vi "py-lv-comm_readInt.vi"(7 "Property":bool, 8 "error in (no error)":errorcluster, 9 "arguments":string[](array[string]), 10 "function":string, 11 "zmq_socket in":refnum<class "zmq_socket.lvclass">) -> (0 "error out":errorcluster, 2 "int result":i32, 3 "zmq_socket out":refnum<class "zmq_socket.lvclass">)   [LabVIEW 2016]
uses:
  <vilib>/addons/zeromq/zmq_socket.lvclass
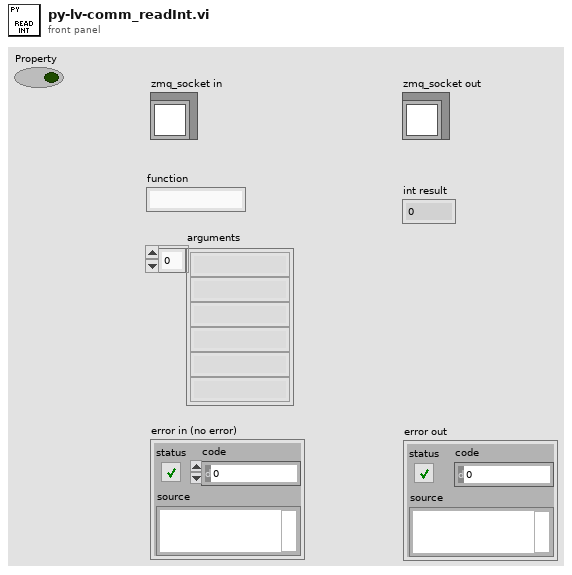
[diagram p1: front panel]
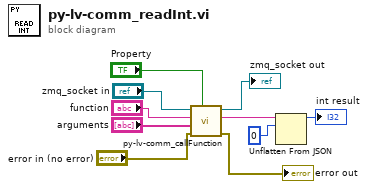
[diagram p0: block diagram]
diagram:
  n1 = call "py-lv-comm_callFunction.vi"("Property (F)"="Property", "error in (no error)"="error in (no error)", "arguments"="arguments", "function"="function", "zmq_socket in"="zmq_socket in") -> ("error out"=→"error out":errorcluster, "return value"=w10:string, "zmq_socket out"=→"zmq_socket out":refnum<class "zmq_socket.lvclass">)  [unwired: 4 in]
  n2 = Unflatten From JSON(JSON string=w10, type and defaults=0) -> (value=→"int result":i32)  [unwired: 5 in, 1 out]
